vi "Voltage - Pressure Amb Conversion.vi"(3 "mean":dbl) -> (7 "Numeric":dbl)   [LabVIEW 2018]
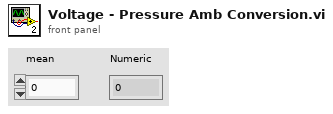
[diagram p1: front panel]
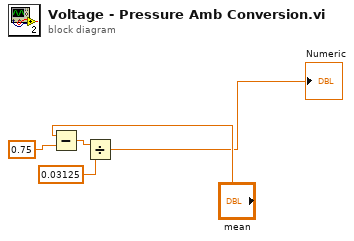
[diagram p0: block diagram]
diagram:
  n1 = Subtract(x="mean", y=0.75 ("minimum value")) -> (x-y=w2:dbl)
  n2 = Divide(x=w2, y=0.03125 ("minimum value")) -> (x/y=→"Numeric":dbl)
